vi "proj 3.vi"() -> ()   [LabVIEW 2022 SP3]
panel:
  in  "Numeric 2":dbl
  in  "Numeric":dbl
  out "Thermometer":dbl(slide) scale=0.0..100.0
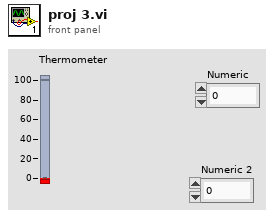
[diagram p1: front panel]
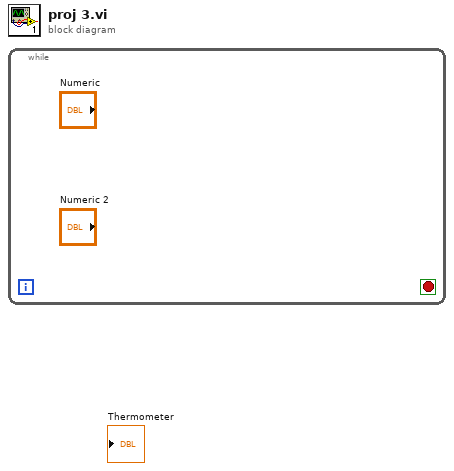
[diagram p0: block diagram]
diagram:
  n1 = while {
    stop <- _ stop-if-true
  }
